vi "LWXPS_GroupHomeSearchAndRelativeMove.vi"(0 "XPS Reference IN":refnum<k24>, 5 "Group Name":string, 7 "Target Displacement IN":dbl[](array[numeric]), 9 "Number of positioners":i32, 11 "LabVIEW error IN":errorcluster) -> (4 "XPS Reference OUT":refnum<k24>, 6 "Returned error code":i32, 8 "Target Displacement OUT":dbl[](array[numeric]), 10 "XPS Error String":string, 15 "LabVIEW error OUT":errorcluster)   [LabVIEW 2014]
uses:
  D:/XPSQ8_LabView_Library/Development/Source/Dll/Newport.XPS.CommandInterface.dll
  Dll/Newport.XPS.CommandInterface.dll
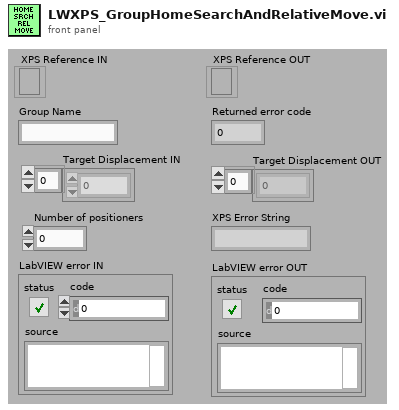
[diagram p1: front panel]
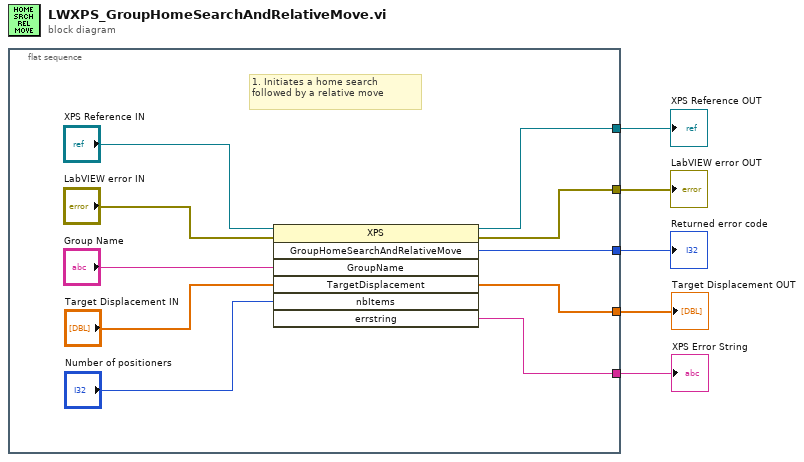
[diagram p0: block diagram]
diagram:
  n1 = flat-sequence {
    tunnel: [w13] -> w5
    tunnel: [w7] -> w4
    tunnel: [w14] -> w3
    tunnel: [w10] -> w1
    tunnel: [w8] -> w2
    frame #0 {
      # "1. Initiates a home search followed by a relative move"
      n2 = invoke class="XPS" method="GroupHomeSearchAndRelativeMove"(reference="XPS Reference IN", error in="LabVIEW error IN", "GroupName"="Group Name", "TargetDisplacement"="Target Displacement IN", "nbItems"="Number of positioners") -> (reference out=w13:refnum<k24>, error out=w7:errorcluster, "GroupHomeSearchAndRelativeMove"=w14:i32, "TargetDisplacement"=w10:dbl[], "errstring"=w8:string)  [unwired: 2 in, 2 out]
    }
  }
  "XPS Reference OUT" <- w5
  "LabVIEW error OUT" <- w4
  "Returned error code" <- w3
  "XPS Error String" <- w2
  "Target Displacement OUT" <- w1
